vi "Create Win Msg Q.vi"(4 "error in (no error)":errorcluster, 5 "Messeges (none)":u32[](array[numeric]) format="%.0x", 7 "VI Refnum":refnum<vi>) -> (0 "error out":errorcluster, 3 "win msg queue":T1)   [LabVIEW 2011]
doc: "Creates a new Windows Message Queue. The queue stores all messages that match any listed in the \"Messages\" input array that are passed to the \"Window Name\" window. The messages can later be retreived from the queue using Wait on Windows Message.vi\n\nParameters:\n\nMessages: The messages that should be queued. For a list of standard windows messages, see the readme file or winuser.h. Default will detect no messages.\n\nWindow Name: Specifies which VI's front panel to monitor. Defaults to the calling VI.\n\nwin msg queue: The new win msg queue refnum.\n\nErrors:\nReturns 6750 if the queue cannot be created."
uses:
  Win Msg Q RefNum.ctl
  lvwinmsg.dll
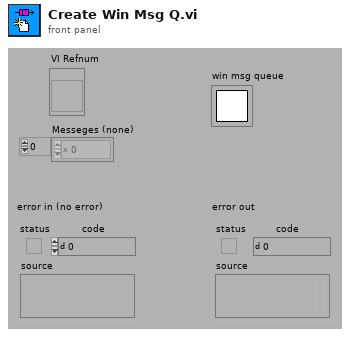
[diagram p1: front panel]
types:
  T1 = typedef "Win Msg Q RefNum.ctl" = refnum<k1>
  T2 = typedef "hWnd.ctl" = refnum<k1>
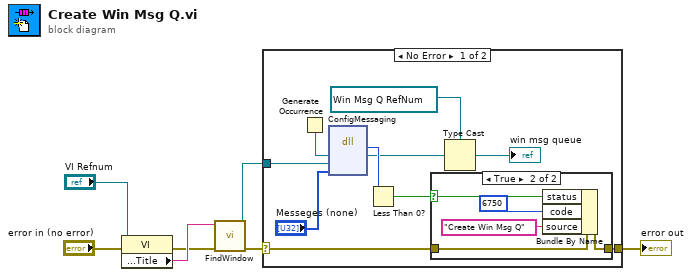
[diagram p0: block diagram]
diagram:
  n1 = property class="VI"(reference="VI Refnum", error in="error in (no error)") -> (error out=w1:errorcluster, "Front Panel Window:Title"=w3:string)  [unwired: 1 out]
  n2 = call "FindWindow.vi"("error in (no error)"=w1, "window name (\"\")"=w3) -> ("error out"=w5:errorcluster, "hWnd"=w6:T2)  [unwired: 6 out]
  n3 = case shown="No Error" w5 {
    selector: w5 -> [w8 w24]
    tunnel: w6 -> [w15 _]
    tunnel: [w12 w24] -> w7
    frame No Error {
      w10 = T1 refnum items=["win msg queue"] ("*(type *) &x")
      n4 = Generate Occurrence() -> (w16:refnum<k4>)
      n5 = dll-call lib="C:/Development/SI.LIB/WIN32/WinMSGQ/lvwinmsg.dll" fn="ConfigMessaging"("occurrence"=w16, "hWnd"=w15, "Messeges (none)"="Messeges (none)") -> (w14:i32, "occurrence"=w11:refnum<k4>)  [unwired: 5 in, 2 out]
      n6 = Less Than 0?(x=w14) -> (x < 0?=w13:bool)
      n7 = case shown="True" w13 {
        selector: w13 -> [_ w19]
        tunnel: w8 -> [w18 w21]
        tunnel: [w18 w20] -> w12
        frame False {
        }
        frame True {
          n8 = Bundle By Name(cluster=w21, "status"=w19, "code"=6750 ("Error Code"), "source"="Create Win Msg Q") -> (w20:errorcluster)
        }
      }
      n9 = Type Cast(type=w10, x=w11) -> (*(type *) &x=→"win msg queue":T1)
    }
    frame Error {
    }
  }
  "error out" <- w7
